vi "Update.vi"(8 "error in (no error)":errorcluster, 11 "SimpleAF in":refnum<class "SimpleAF.lvclass">) -> (0 "error out":errorcluster, 3 "SimpleAF out":refnum<class "SimpleAF.lvclass">)   [LabVIEW 2013]
uses:
  SimpleAF.lvclass
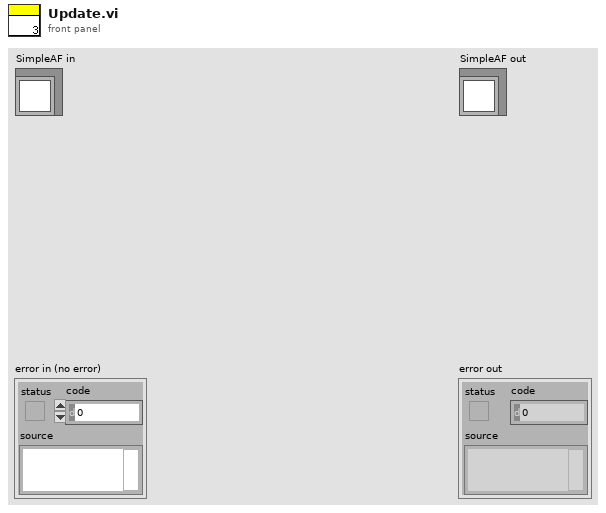
[diagram p1: front panel]
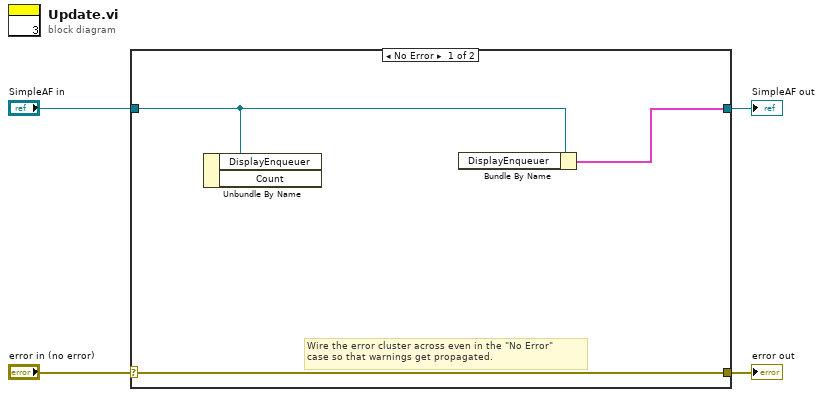
[diagram p0: block diagram]
diagram:
  n1 = case shown="No Error" "error in (no error)" {
    selector: "error in (no error)" -> [w7 w9]
    tunnel: [w7 w9] -> w3
    tunnel: [w5 w8] -> w1
    tunnel: "SimpleAF in" -> [w6 w8]
    frame No Error {
      # "Wire the error cluster across even in the \"No Error\"\ncase so that warnings get propagated."
      n2 = Unbundle By Name(w6) -> ()  [unwired: 2 out]
      n3 = Bundle By Name(cluster=w6) -> (w5:cluster{})  [unwired: 1 in]
    }
    frame Error {
    }
  }
  "error out" <- w3
  "SimpleAF out" <- w1
